vi "PH_Connection.select PCS Node.vi"(5 "error in":errorcluster) -> (16 "string out":string, 19 "error out":errorcluster)   [LabVIEW 2014, in "PH_Common.lvlib"]
doc: "This VI is forseen to select a string from an array of strings."
uses:
  PH_Common.lvlib
panel:
  in  "\"D:\\PCS\\Remote Access\\uOPA.rdp\"":bool caption="uOPA"
  in  "\"D:\\PCS\\Remote Access\\PulsedPower-PA.rdp\"":bool caption="PHPC001"
  in  "\"D:\\PCS\\Remote Access\\Max.rdp\"":bool caption="PHPC001"
  in  "\"D:\\PCS\\Remote Access\\Beckhoff.rdp\"":bool caption="PHPC001"
  in  "\"D:\\PCS\\Remote Access\\PulsedPower-Beckhoff.rdp\"":bool caption="PHPC001"
  in  "ALL ...":bool
  in  "\"D:\\PCS\\Remote Access\\Timing.rdp\"":bool caption="PHPC001"
  in  "\"D:\\PCS\\Remote Access\\Timing-2.rdp\"":bool caption="PHPC001"
  in  "\"D:\\PCS\\Remote Access\\PulsedPower.rdp\"":bool caption="PHPC001"
  in  "\"D:\\PCS\\Remote Access\\Lila.rdp\"":bool caption="PHPC001"
  in  "\"D:\\PCS\\Remote Access\\Global.rdp\"":bool caption="PHPC001"
  in  "\"D:\\PCS\\Remote Access\\Udo.rdp\"":bool caption="PHPC001"
  in  "\"D:\\PCS\\Remote Access\\Christian.rdp\"":bool caption="PHPC001"
  in  "\"D:\\PCS\\Remote Access\\Shotdirector.rdp\"":bool caption="Shot-\ndirector"
  in  "\"D:\\PCS\\Remote Access\\Z6-Compressor.rdp\"":bool caption="Z6 COS"
  in  "\"D:\\PCS\\Remote Access\\Z6-Southtower.rdp\"":bool caption="ST"
  in  "\"D:\\PCS\\Remote Access\\Z6-Northtower.rdp\"":bool caption="NT"
  in  "\"D:\\PCS\\Remote Access\\Laserlabor.rdp\"":bool caption="Exp LL"
  in  "\"D:\\PCS\\Remote Access\\Experiment.rdp\"":bool caption="Exp LB"
  in  "\"D:\\PCS\\Remote Access\\COS.rdp\"":bool caption="COS"
  in  "\"D:\\PCS\\Remote Access\\MAS.rdp\"":bool caption="MAS"
  in  "\"D:\\PCS\\Remote Access\\MA.rdp\"":bool caption="MA"
  in  "\"D:\\PCS\\Remote Access\\PA-Exit.rdp\"":bool caption="PA Exit"
  in  "\"D:\\PCS\\Remote Access\\PA-Input.rdp\"":bool caption="PA Input"
  in  "\"D:\\PCS\\Remote Access\\fs.rdp\"":bool caption="fs FE"
  in  "\"D:\\PCS\\Remote Access\\ns.rdp\"":bool caption="ns FE"
  in  "Cancel":bool
  # "PCS"
  # "3.40"
  # "Exp 4: Z6"
  # "Beam Diag.\nPLH 2.002"
  # "ELT  PLH 2.004"
  # "Laser Labor\nPLH 1.001"
  # "Test Labor\nPLH 2.001"
  # "Stairway"
  # "Stairway"
  # "Laser Bay\nPLH 1.002"
  # "PKR\nPLH 2.007"
  # "HV Room\nPLH 2.005"
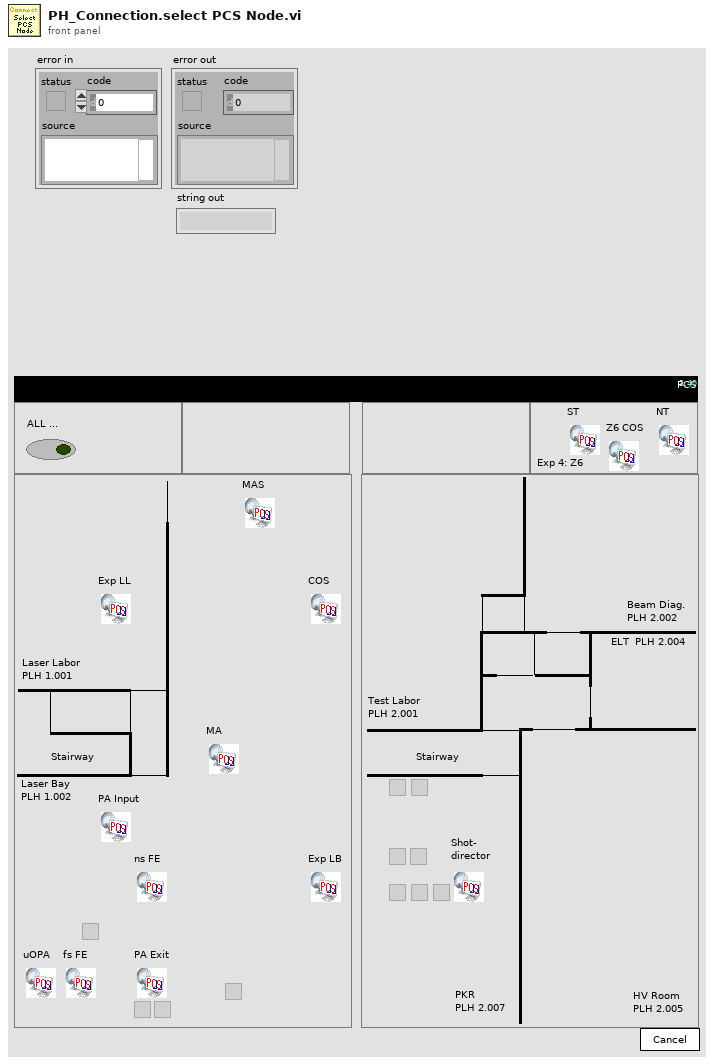
[diagram p1: front panel]
types:
  T1 = enum8{"Enabled", "Disabled", "Disabled and Grayed Out"}
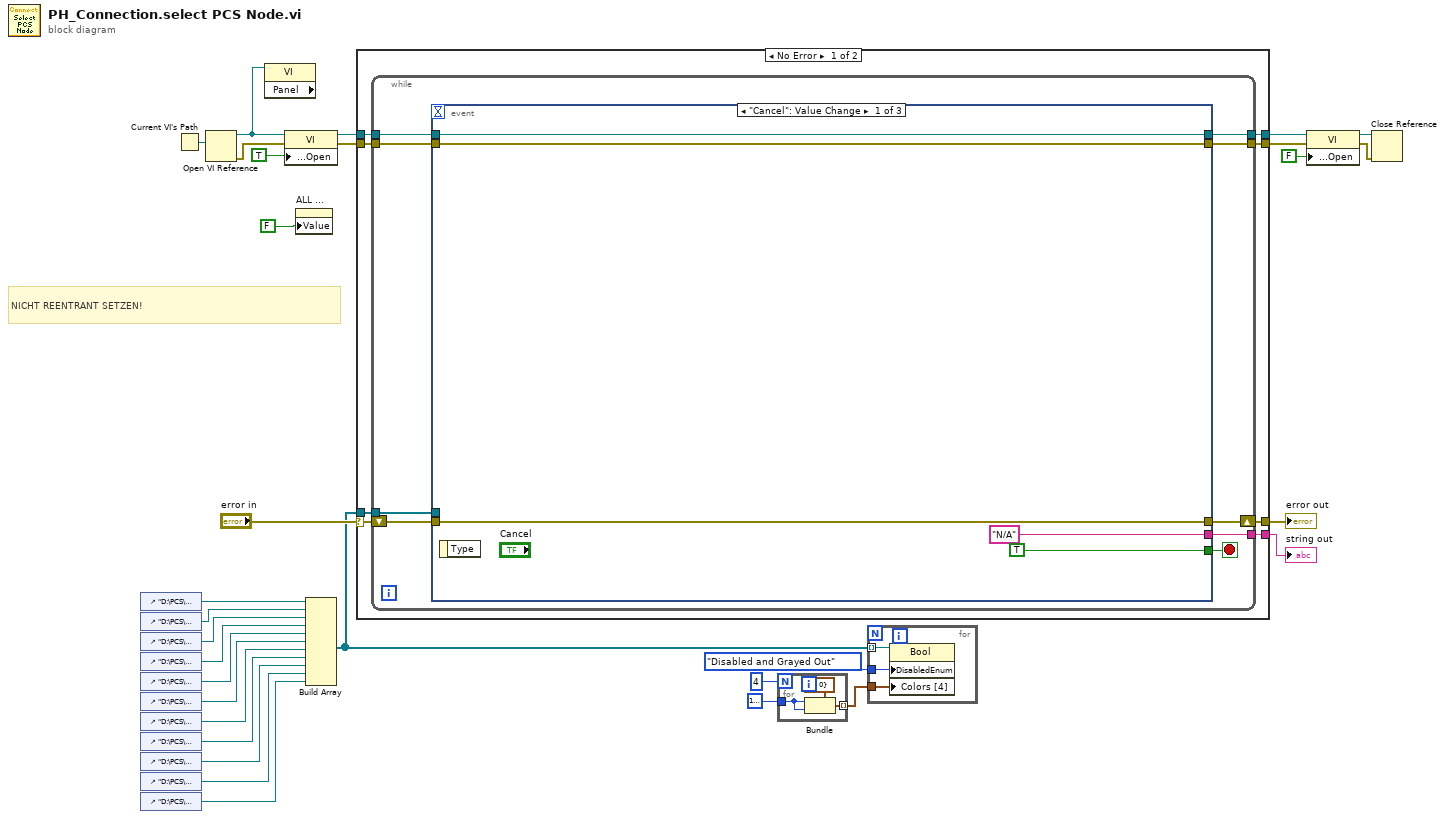
[diagram p0: block diagram]
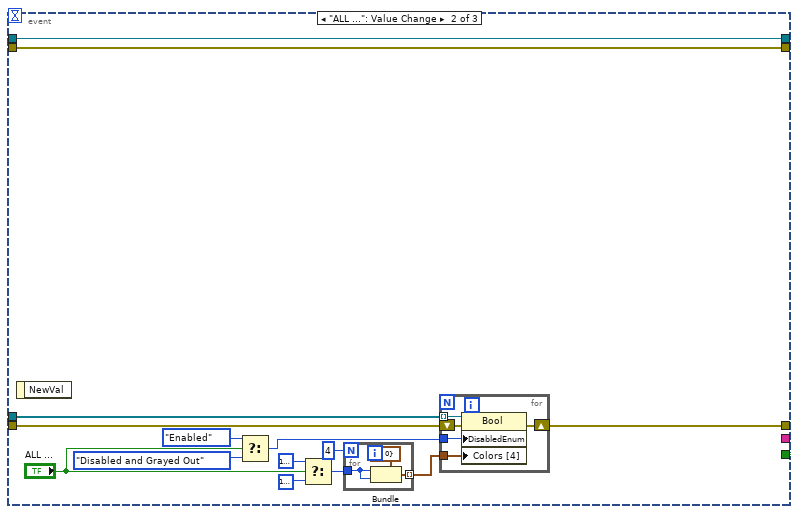
[diagram p2: hidden frame]
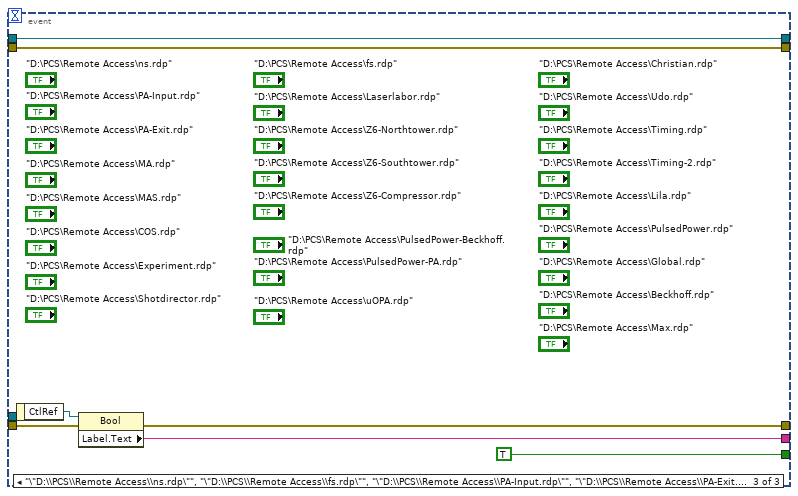
[diagram p3: hidden frame]
diagram:
  # "NICHT REENTRANT SETZEN!"
  n1 = control-ref of="\"D:\\PCS\\Remote Access\\Christian.rdp\""() -> (w19:refnum<vi>)
  n2 = control-ref of="\"D:\\PCS\\Remote Access\\Udo.rdp\""() -> (w18:refnum<vi>)
  n3 = control-ref of="\"D:\\PCS\\Remote Access\\PulsedPower-PA.rdp\""() -> (w17:refnum<vi>)
  n4 = control-ref of="\"D:\\PCS\\Remote Access\\Timing.rdp\""() -> (w16:refnum<vi>)
  n5 = control-ref of="\"D:\\PCS\\Remote Access\\Timing-2.rdp\""() -> (w15:refnum<vi>)
  n6 = control-ref of="\"D:\\PCS\\Remote Access\\PulsedPower-Beckhoff.rdp\""() -> (w14:refnum<vi>)
  n7 = control-ref of="\"D:\\PCS\\Remote Access\\Lila.rdp\""() -> (w13:refnum<vi>)
  n8 = control-ref of="\"D:\\PCS\\Remote Access\\PulsedPower.rdp\""() -> (w12:refnum<vi>)
  n9 = control-ref of="\"D:\\PCS\\Remote Access\\Max.rdp\""() -> (w11:refnum<vi>)
  n10 = control-ref of="\"D:\\PCS\\Remote Access\\Global.rdp\""() -> (w10:refnum<vi>)
  n11 = control-ref of="\"D:\\PCS\\Remote Access\\Beckhoff.rdp\""() -> (w9:refnum<vi>)
  n12 = Current VI's Path() -> (path=w28:path)
  n13 = Open VI Reference(vi path=w28) -> (vi reference=w1:refnum<vi>, error out=w22:errorcluster)  [unwired: 5 in]
  n14 = property class="VI" props=["Panel"](reference=w1) -> ()  [unwired: 1 in, 3 out]
  n15 = property class="VI"(reference=w1, error in=w22, "Front Panel Window:Open"=TRUE) -> (reference out=w26:refnum<vi>, error out=w8:errorcluster)
  n16 = property on="ALL ..." class="Bool (strict)"("Value"=FALSE ("ALL ...")) -> ()  [unwired: 2 in, 2 out]
  n17 = Build Array(w19, w18, w17, w16, w15, w14, w13, w12, w11, w10, w9) -> (w6:refnum<vi>[])
  n18 = case shown="No Error" "error in" {
    selector: "error in" -> [w35 w87]
    tunnel: [w39 "N/A" ("String")] -> w31
    tunnel: [w36 w87] -> w30
    tunnel: w26 -> [w38 w86]
    tunnel: [w37 w86] -> w24
    tunnel: w6 -> [w34 _]
    tunnel: w8 -> [w33 w84]
    tunnel: [w32 w84] -> w7
    frame No Error {
      n19 = while {
        tunnel: [w48] -> w39
        tunnel: w38 -> [w47]
        tunnel: [w46] -> w37
        shift-right: [w45] -> w36
        shift-left: w35 -> [w44]
        tunnel: w34 -> [w42]
        tunnel: w33 -> [w41]
        tunnel: [w40] -> w32
        stop <- w43 stop-if-true
        n20 = event shown="[0] \"Cancel\": Value Change" {
          selector: _ -> [_ _ _]
          dyn-events: _ -> [_ _ _]
          timeout: _ -> [_ _ _]
          tunnel: ["N/A" ("String") _ w79] -> w48
          tunnel: [w53 w66 w83] -> w46
          tunnel: w47 -> [w53 w66 w83]
          tunnel: w44 -> [w51 w67 w81]
          tunnel: [w51 w64 w78] -> w45
          tunnel: [TRUE FALSE TRUE] -> w43
          tunnel: w42 -> [_ w63 _]
          tunnel: w41 -> [w49 w54 w77]
          tunnel: [w49 w54 w77] -> w40
          event "Cancel": Value Change {
            n21 = event-data() -> ()  [unwired: 1 in, 1 out]
          }
          event "ALL ...": Value Change {
            n22 = event-data() -> ()  [unwired: 1 in, 1 out]
            n23 = Select(t=T1."Enabled" ("Disabled"), s="ALL ...", f=T1."Disabled and Grayed Out" ("Disabled")) -> (s? t:f=w55:T1)
            n24 = Select(t=u32 16777216 ("Color Box"), s="ALL ...", f=u32 16777238 ("Color Box")) -> (s? t:f=w56:u32)
            n25 = for {
              N: 4 -> [_]
              tunnel: w56 -> [w75]
              tunnel: [w74] -> w62 mode=indexing
              n26 = Bundle(cluster=cluster{u32, u32} {0, 0}, w75, w75) -> (w74:cluster{u32, u32})
            }
            n27 = for {
              shift-right: [w72] -> w64
              shift-left: w67 -> [w73]
              tunnel: w63 -> [w71] mode=indexing
              tunnel: w62 -> [w70]
              tunnel: w55 -> [w69]
              n28 = property class="Bool"(reference=w71, error in=w73, "DisabledEnum"=w69, "Colors [4]"=w70) -> (error out=w72:errorcluster)  [unwired: 1 out]
            }
          }
          event "\"D:\\PCS\\Remote Access\\ns.rdp\"", "\"D:\\PCS\\Remote Access\\fs.rdp\"", "\"D:\\PCS\\Remote Access\\PA-Input.rdp\"", "\"D:\\PCS\\Remote Access\\PA-Exit.rdp\"", "\"D:\\PCS\\Remote Access\\MA.rdp\"", "\"D:\\PCS\\Remote Access\\MAS.rdp\"", "\"D:\\PCS\\Remote Access\\COS.rdp\"", "\"D:\\PCS\\Remote Access\\Experiment.rdp\"", "\"D:\\PCS\\Remote Access\\Laserlabor.rdp\"", "\"D:\\PCS\\Remote Access\\Z6-Northtower.rdp\"", "\"D:\\PCS\\Remote Access\\Z6-Southtower.rdp\"", "\"D:\\PCS\\Remote Access\\Z6-Compressor.rdp\"", "\"D:\\PCS\\Remote Access\\Shotdirector.rdp\"", "\"D:\\PCS\\Remote Access\\Christian.rdp\"", "\"D:\\PCS\\Remote Access\\Udo.rdp\"", "\"D:\\PCS\\Remote Access\\Global.rdp\"", "\"D:\\PCS\\Remote Access\\Lila.rdp\"", "\"D:\\PCS\\Remote Access\\PulsedPower.rdp\"", "\"D:\\PCS\\Remote Access\\Timing-2.rdp\"", "\"D:\\PCS\\Remote Access\\Timing.rdp\"", "\"D:\\PCS\\Remote Access\\PulsedPower-Beckhoff.rdp\"", "\"D:\\PCS\\Remote Access\\Beckhoff.rdp\"", "\"D:\\PCS\\Remote Access\\Max.rdp\"", "\"D:\\PCS\\Remote Access\\PulsedPower-PA.rdp\"", "\"D:\\PCS\\Remote Access\\uOPA.rdp\"": Value Change {
            n29 = event-data() -> ("CtlRef"=w82:refnum<vi>)  [unwired: 1 in]
            n30 = property class="Bool"(reference=w82, error in=w81) -> (error out=w78:errorcluster, "Label.Text"=w79:string)  [unwired: 1 out]
          }
        }
      }
    }
    frame Error {
    }
  }
  "error out" <- w30
  "string out" <- w31
  n31 = for {
    N: 4 -> [_]
    tunnel: u32 16777238 ("Color Box") -> [w89]
    tunnel: [w88] -> w2 mode=indexing
    n32 = Bundle(cluster=cluster{u32, u32} {0, 0}, w89, w89) -> (w88:cluster{u32, u32})
  }
  n33 = for {
    tunnel: w6 -> [w93] mode=indexing
    tunnel: w2 -> [w92]
    tunnel: T1."Disabled and Grayed Out" ("Disabled") -> [w91]
    n34 = property class="Bool"(reference=w93, "DisabledEnum"=w91, "Colors [4]"=w92) -> ()  [unwired: 1 in, 2 out]
  }
  n35 = property class="VI"(reference=w24, error in=w7, "Front Panel Window:Open"=FALSE) -> (reference out=w23:refnum<vi>, error out=w21:errorcluster)
  n36 = Close Reference(reference=w23, error in (no error)=w21) -> ()  [unwired: 1 out]
